vi "Apply Digital In Names.vi"(8 "error in (no error)":errorcluster, 11 "DAQ970 in":refnum<class "DAQ970.lvclass">) -> (0 "error out":errorcluster, 3 "DAQ970 out":refnum<class "DAQ970.lvclass">)   [LabVIEW 2019, in "DAQ970.lvlib" / "DAQ970.lvclass"]
uses:
  Library/DAQ970.lvclass
  Library/DAQ970.lvclass/DAQ970.ctl
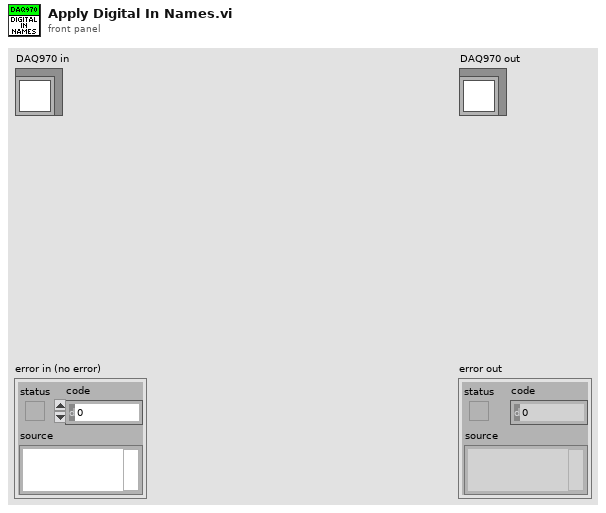
[diagram p1: front panel]
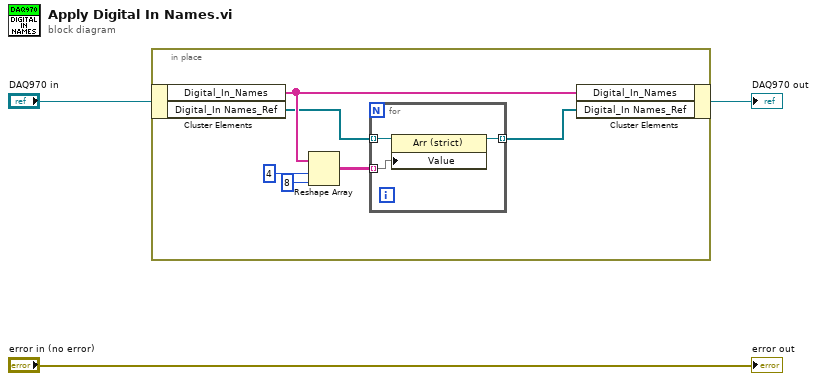
[diagram p0: block diagram]
diagram:
  n1 = in-place {
    n2 = in-place-cluster #1("DAQ970 in") -> ("Digital_In_Names"=w9:string[], "Digital_In Names_Ref"=w6:refnum<vi>[])
    n3 = Reshape Array(w9, 4 ("dimension size"), 8 ("dimension size")) -> (w4:string[][])
    n4 = for {
      tunnel: w6 -> [w12] mode=indexing
      tunnel: [w11] -> w5 mode=indexing
      tunnel: w4 -> [w10] mode=indexing
      n5 = property class="Arr (strict)"(reference=w12, "Value"=w10) -> (reference out=w11:refnum<vi>)  [unwired: 1 in, 1 out]
    }
    n6 = in-place-cluster #1("Digital_In_Names"=w9, "Digital_In Names_Ref"=w5) -> (→"DAQ970 out":refnum<class "DAQ970.lvclass">)
  }
  "error out" <- "error in (no error)"
